vi "DisplaySquare.vi"(6 "square":T1, 7 "Grid":T2, 8 "new picture in":picture) -> (5 "new picture out":picture)   [LabVIEW 2020]
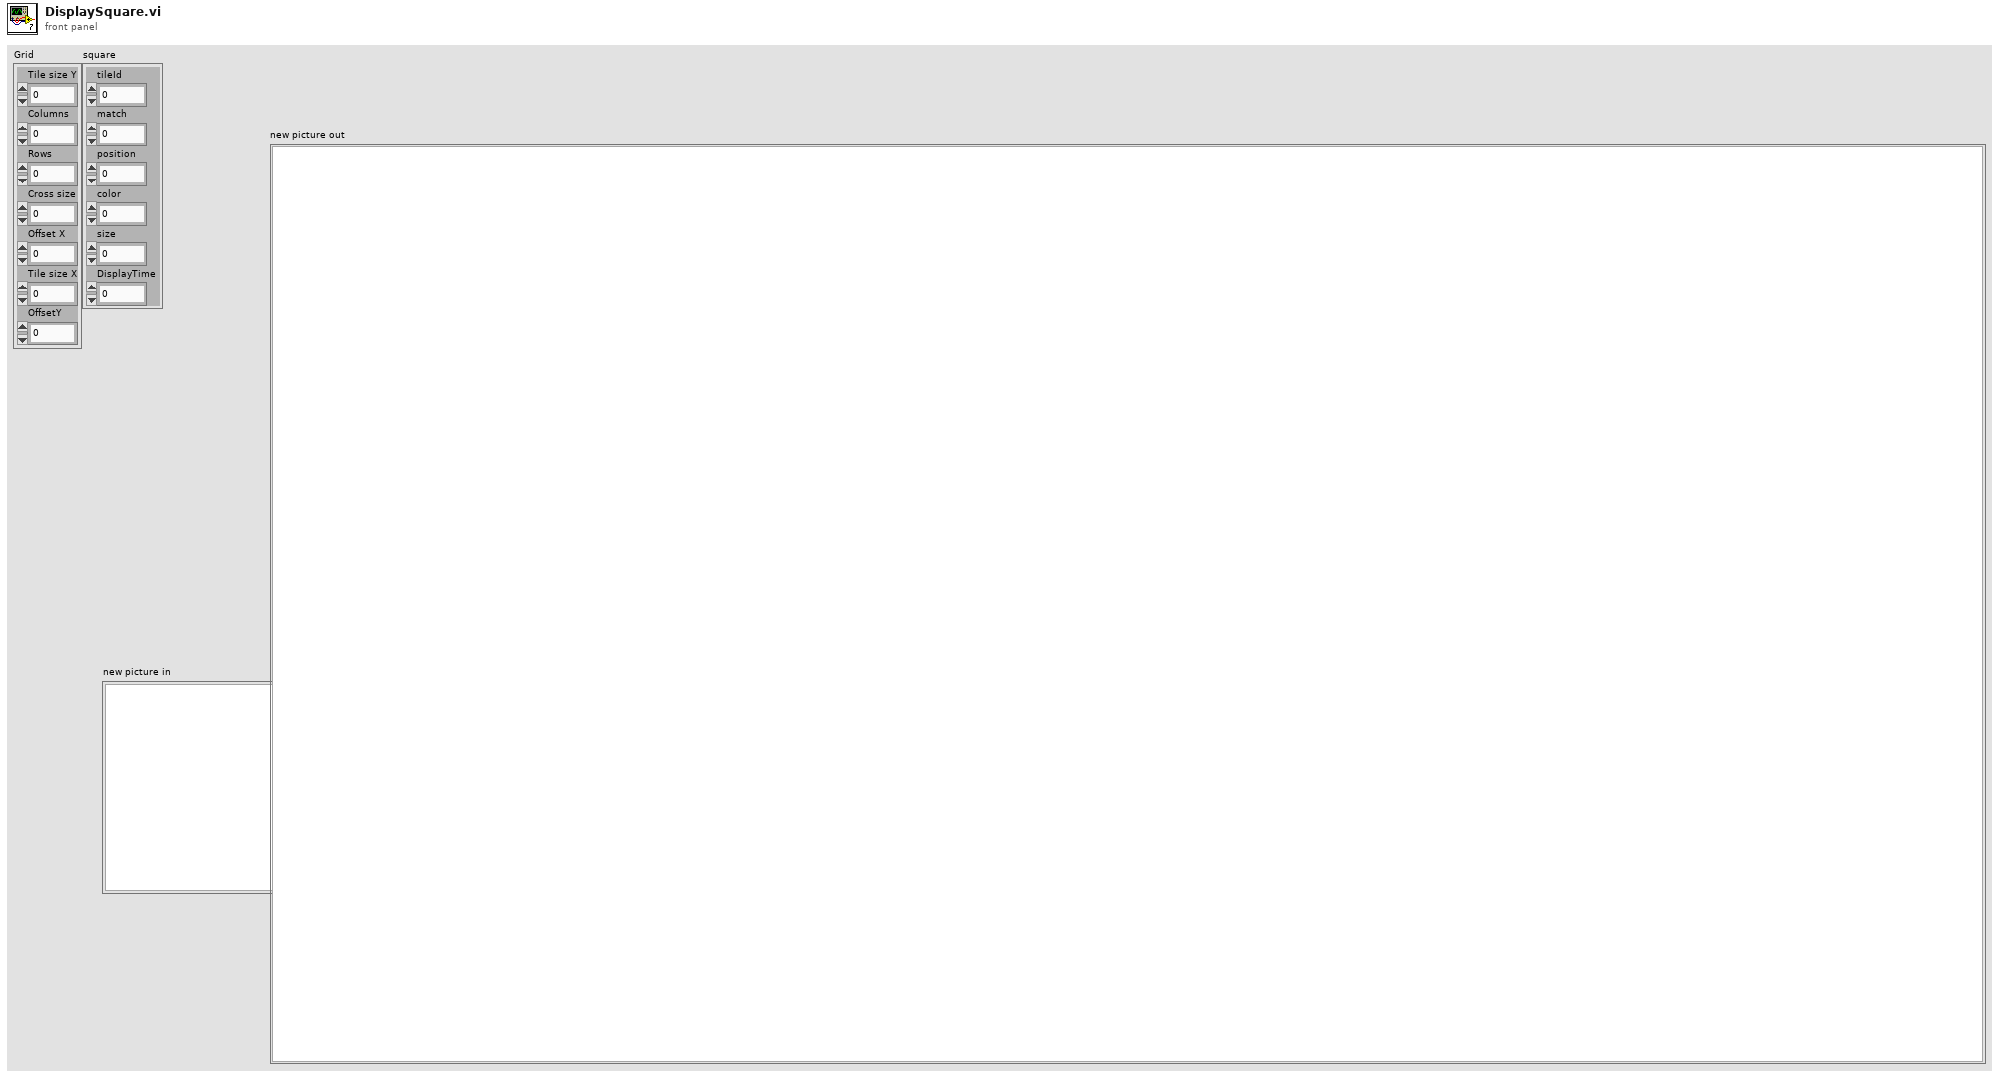
[diagram p1: front panel]
types:
  T1 = cluster{"tileId":i32, "match":i32, "position":i32, "color":u32, "size":i32, "DisplayTime":i32}
  T2 = cluster{"Tile size Y":dbl, "Columns":dbl, "Rows":dbl, "Cross size":dbl, "Offset X":dbl, "Tile size X":dbl, "OffsetY":dbl}
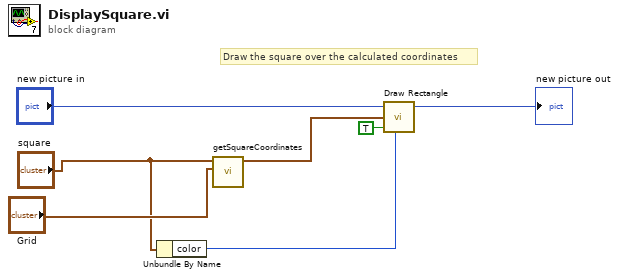
[diagram p0: block diagram]
diagram:
  # "Draw the square over the calculated coordinates"
  n1 = Unbundle By Name("square") -> ("color"=w3:u32)
  n2 = call "getSquareCoordinates.vi"("Grid"="Grid", "square"="square") -> ("Cluster"=w6:cluster{dbl, dbl, dbl, dbl})  [unwired: 9 in]
  n3 = call <vilib>:"Draw Rectangle.vi"("picture"="new picture in", "rect"=w6, "fill?(F)"=TRUE, "color(black)"=w3) -> ("new picture"=→"new picture out":picture)  [unwired: 5 in]
